vi "File to Gcode.vi"(11 "File Path":path) -> (3 "G-Code Array":string[](array[string]))   [LabVIEW 2021]
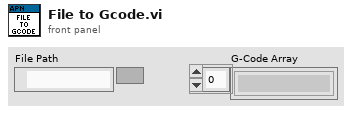
[diagram p1: front panel]
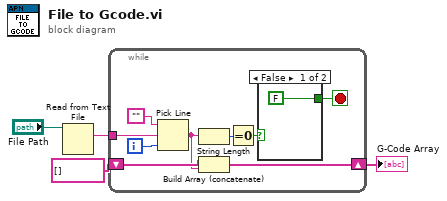
[diagram p0: block diagram]
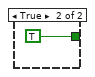
[diagram p2: hidden frame]
diagram:
  n1 = Read from Text File(file (use dialog)="File Path") -> (text=w2:string)  [unwired: 3 in, 3 out]
  n2 = while {
    shift-right: [w11] -> w3
    shift-left: string[] [] -> [w12]
    tunnel: w2 -> [w6]
    i -> [w13]
    stop <- w5 stop-if-true
    n3 = Pick Line(string ("")="", multi-line string=w6, line index=w13) -> (output string=w9:string)
    n4 = String Length(string=w9) -> (length=w8:i32)
    n5 = Build Array (concatenate)(w12, w9) -> (w11:string[])
    n6 = Equal To 0?(x=w8) -> (x = 0?=w7:bool)
    n7 = case shown="False" w7 {
      tunnel: [FALSE TRUE] -> w5
      frame False {
      }
      frame True {
      }
    }
  }
  "G-Code Array" <- w3
